vi "PM100D_ConfMeas.vi"(2 "error in":errorcluster, 3 "Conf:":string(combo)="POW", 4 "VISA In":refnum<visa-resource-name>) -> (0 "error out":errorcluster, 1 "dup VISA session":refnum<visa-resource-name>)   [LabVIEW 2012]
doc: "- Configure measurement with SCPI command CONF:POW\n- ABORt measurement\n- Clear operation register with STAT:OPER?\n- INITialize measurement"
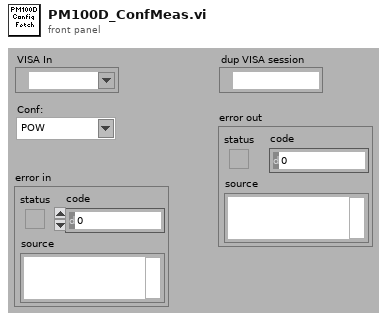
[diagram p1: front panel]
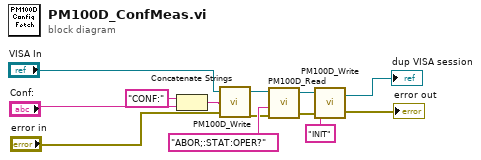
[diagram p0: block diagram]
diagram:
  n1 = Concatenate Strings("CONF:" ("string"), "Conf:") -> (w4:string)
  n2 = call "PM100D_Write.vi"("error in (no error)"="error in", "Command"=w4, "VISA in"="VISA In") -> ("error out"=w9:errorcluster, "VISA out"=w7:refnum<visa-resource-name>)
  n3 = call "PM100D_Read.vi"("error in (no error)"=w9, "Command"="ABOR;:STAT:OPER?", "VISA in"=w7) -> ("error out"=w10:errorcluster, "VISA out"=w8:refnum<visa-resource-name>)  [unwired: 1 in, 1 out]
  n4 = call "PM100D_Write.vi"("error in (no error)"=w10, "Command"="INIT", "VISA in"=w8) -> ("error out"=→"error out":errorcluster, "VISA out"=→"dup VISA session":refnum<visa-resource-name>)
